vi "GetRoutes.vi"(8 "error in (no error)":errorcluster, 11 "reference in":refnum<class "Switch_MotorP5.lvclass">) -> (0 "error out":errorcluster, 2 "Routes":T1(array[cluster]), 3 "reference in":refnum<class "Switch_MotorP5.lvclass">)   [LabVIEW 2022 SP3, in "Switch_MotorP5.lvlib" / "Switch_MotorP5.lvclass"]
uses:
  Switch_MotorP5.lvclass
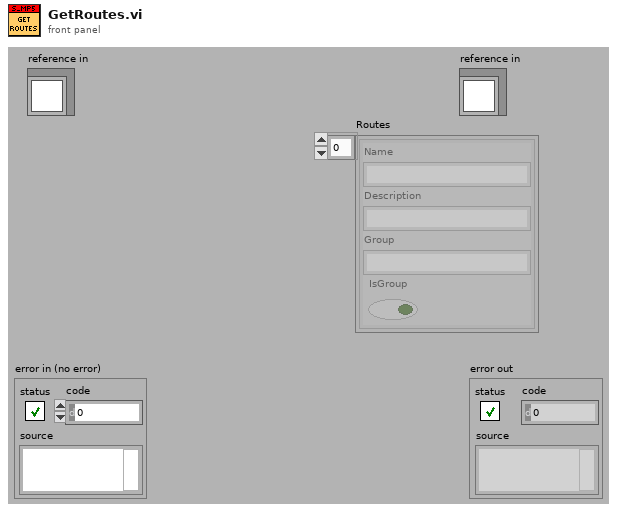
[diagram p1: front panel]
types:
  T1 = cluster{"Name":string, "Description":string, "Group":string, "IsGroup":bool}[]
  T2 = cluster{"Name":string, "Description":string, "Group":string, "IsGroup":bool}
  T3 = typedef "Switch_MotorP5.lvlib/Switch_MotorP5.lvclass/ObjectAttributes.ctl" = cluster{"Config":T4, "VISA":refnum<visa-resource-name>, "RPM":i32, "States":bool[], "UpdateEvent":refnum<user-event>, "Motor":enum32{"M1", "M2", "M3", "M4", "M5", "M6", "M7", "M8"}}
  T4 = typedef "Switch_MotorP5.lvlib/Switch_MotorP5.lvclass/Config.ctl" = cluster{"COM":refnum<visa-resource-name>, "SwitchMap":cluster{"Name":string, "Description":string, "Group":string, "IsGroup":bool, "Motor":enum32{"M1", "M2", "M3", "M4", "M5", "M6", "M7", "M8", "NA"}}[], "Sim":bool}
  T5 = cluster{"Name":string, "Description":string, "Group":string, "IsGroup":bool, "Motor":enum32{"M1", "M2", "M3", "M4", "M5", "M6", "M7", "M8", "NA"}}[]
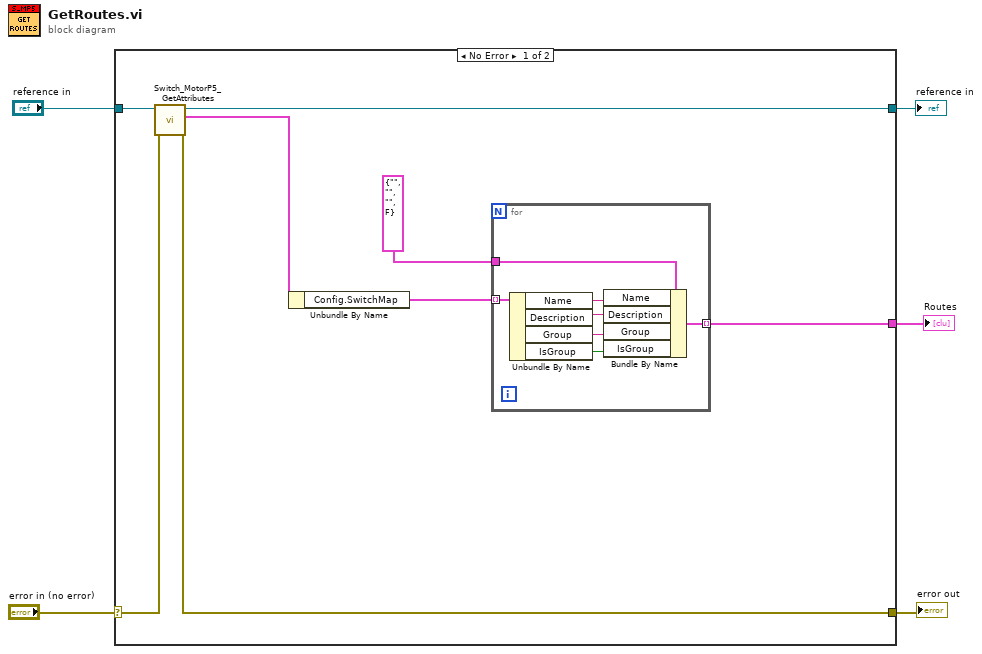
[diagram p0: block diagram]
diagram:
  n1 = case shown="No Error" "error in (no error)" {
    selector: "error in (no error)" -> [w13 w22]
    tunnel: [w11 w22] -> w4
    tunnel: [w9 w21] -> w2
    tunnel: "reference in" -> [w10 w21]
    tunnel: [w6 _] -> w1
    frame No Error {
      n2 = call "Switch_MotorP5_GetAttributes.vi"("error in (no error)"=w13, "reference in"=w10) -> ("error out"=w11:errorcluster, "Data"=w12:T3, "reference out"=w9:refnum<class "Switch_MotorP5.lvclass">)  [unwired: 6 in, 1 out]
      n3 = Unbundle By Name(w12) -> ("Config.SwitchMap"=w8:T5)
      n4 = for {
        tunnel: w8 -> [w20] mode=indexing
        tunnel: T2 {"Name"="", "Description"="", "Group"="", "IsGroup"=FALSE} ("Route") -> [w18]
        tunnel: [w14] -> w6 mode=indexing
        n5 = Unbundle By Name(w20) -> ("Name"=w19:string, "Description"=w17:string, "Group"=w16:string, "IsGroup"=w15:bool)
        n6 = Bundle By Name(cluster=w18, "Name"=w19, "Description"=w17, "Group"=w16, "IsGroup"=w15) -> (w14:T2)
      }
    }
    frame Error {
    }
  }
  "error out" <- w4
  "reference in" <- w2
  "Routes" <- w1
